vi "Float Precision.vi"(8 "Enum":enum16{"Set", "Get"}(ring), 11 "Precision":u8=6) -> (0 "Format String":string, 3 "Precision out":u8)   [LabVIEW 2017, in "API String Arguments Support.lvlib"]
uses:
  API String Arguments Support.lvlib
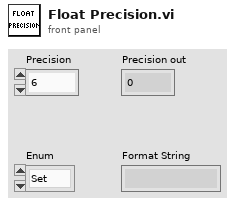
[diagram p1: front panel]
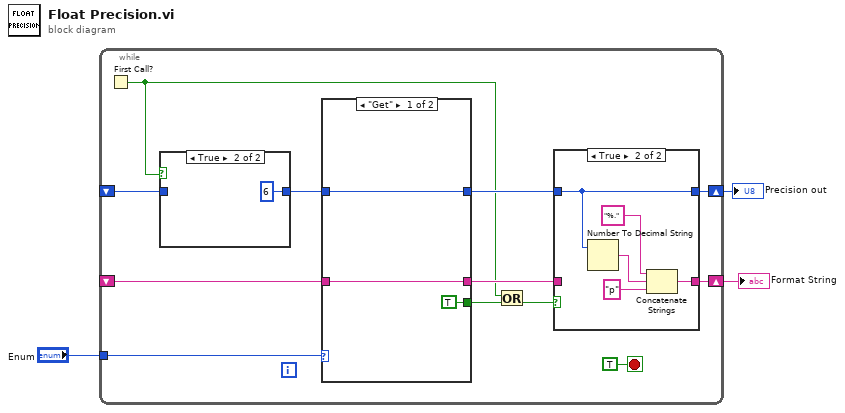
[diagram p0: block diagram]
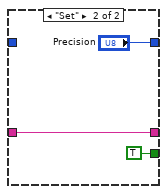
[diagram p3: hidden frame]
diagram:
  n1 = while {
    tunnel: "Enum" -> [w14]
    shift-right: [w13] -> w2
    shift-left: _ -> [w12]
    shift-right: [w8] -> w1
    shift-left: _ -> [w4]
    stop <- TRUE stop-if-true
    n2 = First Call?() -> (First Call?: T/F=w6:bool)
    n3 = case shown="True" w6 {
      tunnel: [w16 u8 6 ("Precision")] -> w5
      tunnel: w4 -> [w16 _]
      frame False {
      }
      frame True {
      }
    }
    n4 = case shown="\"Get\"" w14 {
      tunnel: w12 -> [w20 w23]
      tunnel: [w20 w23] -> w11
      tunnel: [TRUE TRUE] -> w10
      tunnel: w5 -> [w18 _]
      tunnel: [w18 "Precision"] -> w7
      frame "Get" {
      }
      frame "Set" {
      }
    }
    n5 = Or(x=w6, y=w10) -> (x .or. y?=w9:bool)
    n6 = case shown="True" w9 {
      tunnel: [w25 w27] -> w13
      tunnel: w11 -> [w25 _]
      tunnel: [w24 w26] -> w8
      tunnel: w7 -> [w24 w26]
      frame False {
      }
      frame True {
        n7 = Number To Decimal String(number=w26) -> (decimal integer string=w30:string)  [unwired: 1 in]
        n8 = Concatenate Strings("%." ("format string"), w30, "p" ("format string")) -> (w27:string)
      }
    }
  }
  "Format String" <- w2
  "Precision out" <- w1
